vi "read controls indices.vi"(8 "error in (no error)":errorcluster, 10 "labels":string[](array[string]), 11 "id":string) -> (0 "error out":errorcluster, 2 "indices":i32[](array[numeric]))   [LabVIEW 2024, in "controls manager.lvlib"]
uses:
  controls manager.lvlib
  fgv actions.ctl
  <vilib>/Utility/error.llb/Error Cluster From Error Code.vi
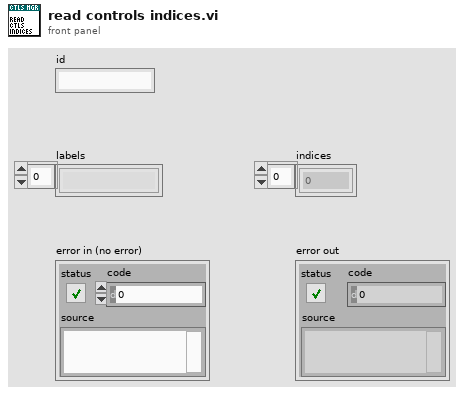
[diagram p1: front panel]
types:
  T1 = typedef "controls manager.lvlib/fgv actions.ctl" = enum16{"create", "get", "destroy"}
  T2 = typedef "controls manager.lvlib/collection type.ctl" = map{string, T3}
  T3 = typedef "controls manager.lvlib/entry type.ctl" = cluster{"controls":map{string, T4}, "plan":T5}
  T4 = typedef "controls manager.lvlib/control.ctl" = cluster{"refnum":refnum<vi>, "index":i32}
  T5 = typedef "controls manager.lvlib/controls plan.ctl" = map{string, T6[]}
  T6 = typedef "controls manager.lvlib/key value pair.ctl" = cluster{"key":string, "value":string}
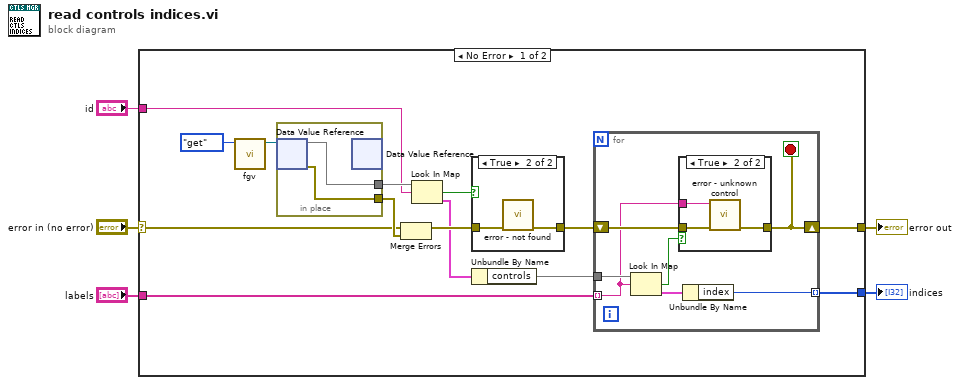
[diagram p0: block diagram]
diagram:
  n1 = case shown="No Error" "error in (no error)" {
    selector: "error in (no error)" -> [w16 w36]
    tunnel: [w8 w36] -> w1
    tunnel: "id" -> [w14 _]
    tunnel: "labels" -> [w6 _]
    tunnel: [w7 _] -> w2
    frame No Error {
      n2 = call "fgv.vi"("action"=fgv_actions."get") -> ("dvr"=w19:refnum<data-value>)  [unwired: 9 in, 1 out]
      n3 = in-place {
        in-place-border: [w24] -> w15
        in-place-border: [w23] -> w17
        n4 = in-place-dvr #1(w19) -> (w24:T2, w23:errorcluster)
        n5 = in-place-dvr #1() -> ()  [unwired: 1 in, 2 out]
      }
      n6 = Merge Errors(w16, w17) -> (w12:errorcluster)
      n7 = Look In Map(map=w15, key=w14) -> (key not found?=w13:bool, value=w11:T3)  [unwired: 1 in]
      n8 = case shown="True" w13 {
        tunnel: w12 -> [w20 w22]
        tunnel: [w20 w21] -> w9
        frame False {
        }
        frame True {
          n9 = call "error - not found.vi"("error in (no error)"=w22) -> ("error out"=w21:errorcluster)  [unwired: 10 in]
        }
      }
      n10 = Unbundle By Name(w11) -> ("controls"=w10:map{string, T4})
      n11 = for {
        tunnel: w10 -> [w31]
        tunnel: [w29] -> w7 mode=indexing
        tunnel: w6 -> [w25] mode=indexing
        shift-right: [w26] -> w8
        shift-left: w9 -> [w28]
        stop <- w26 stop-if-true
        n12 = Look In Map(map=w31, key=w25) -> (key not found?=w27:bool, value=w30:T4)  [unwired: 1 in]
        n13 = case shown="True" w27 {
          tunnel: w28 -> [w32 w35]
          tunnel: [w32 w34] -> w26
          tunnel: w25 -> [_ w33]
          frame False {
          }
          frame True {
            n14 = call "error - unknown control.vi"("error in (no error)"=w35, "label"=w33) -> ("error out"=w34:errorcluster)  [unwired: 9 in]
          }
        }
        n15 = Unbundle By Name(w30) -> ("index"=w29:i32)
      }
    }
    frame Error {
    }
  }
  "error out" <- w1
  "indices" <- w2
